vi "External Control (Example VI).vi"() -> ()   [LabVIEW 2016]
panel:
  in  "Boolean":bool
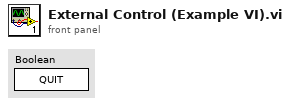
[diagram p1: front panel]
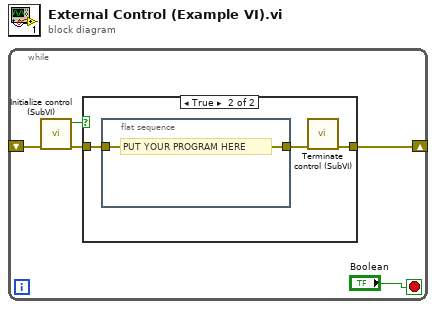
[diagram p0: block diagram]
diagram:
  n1 = while {
    shift-right: [w1] -> _
    shift-left: _ -> [w2]
    stop <- "Boolean" stop-if-true
    n2 = call "Initialize control (SubVI).vi"("error in (no error)"=w2) -> ("error out"=w3:errorcluster, "Control taken?"=w4:bool)  [unwired: 9 in]
    n3 = case shown="True" w4 {
      tunnel: w3 -> [w6 w9]
      tunnel: [w6 w7] -> w1
      frame False {
      }
      frame True {
        n4 = flat-sequence "Put your program here" {
          tunnel: [w10] -> w8
          tunnel: w9 -> [w10]
          frame #0 {
            # "PUT YOUR PROGRAM HERE"
          }
        }
        n5 = call "Terminate control (SubVI).vi"("errorin"=w8) -> ("error out"=w7:errorcluster)  [unwired: 10 in]
      }
    }
  }
